vi "DAQ_OPC UA.vi"() -> (0 "Error Out":errorcluster)   [LabVIEW 2017]
uses:
  <vilib>/dex/Flush And Wait Empty Condition.ctl
  <vilib>/Platform/TimedLoop/XDataNode/timing_clust.ctl
  <vilib>/Platform/TimedLoop/XDataNode/nitl_modes.ctl
  <vilib>/Platform/TimedLoop/XDataNode/wakeup.ctl
  <vilib>/DAQmx/read.llb/DAQmx Read (Analog 1D DBL NChan 1Samp).vi
  <vilib>/DAQmx/miscellaneous.llb/DAQmx Fill In Error Info.vi
  <vilib>/Platform/TimedLoop/XDataNode/XDataNode.xnode
  <vilib>/Platform/TimedLoop/XDataNode/XDNodeRunTimeDep.lvlib
  <resource>/objmgr/ni.dex.rc
panel:
  out "Producer Loop Time":i64
  out "Consumer Loop Time":u32
  out "Time":dbl
  out "Available Elements for Writing":i32
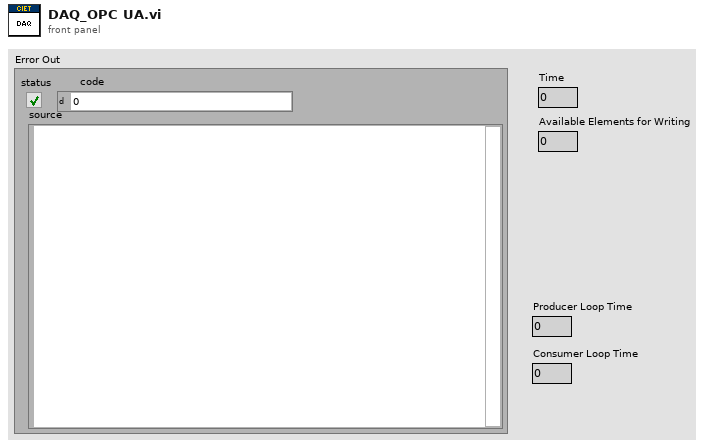
[diagram p1: front panel]
types:
  T1 = typedef "Flush And Wait Empty Condition.ctl" = u8
  T2 = typedef "XDNodeRunTimeDep.lvlib/timing_clust.ctl" = cluster{"Expected End [f-1]":u64, "Actual End [f-1]":u64, "Finished Late? [f-1]":bool, "Expected End [i-1]":u64, "Actual End [i-1]":u64, "Finished Late? [i-1]":bool, "Expected Start [i]":u64, "Actual Start [i]":u64, "Expected Start [f]":u64, "Actual Start [f]":u64, "Source Name":string, "Structure Name":string, "Period":i64, "Deadline":i64, "Offset":i64, "Start":i64, "Priority":i32, "Timeout":i32, "Mode":T3, "Wakeup Reason":T4, "Error":errorcluster, "Source Type":string, "Secondary Source Type":string, "Global End Time":u64, "Global Start Time":u64, "Frame Duration":u64, "Iteration Duration":u64, "Assigned CPU":i32, "I/O Scan Engine Mode":u32}
  T3 = typedef "XDNodeRunTimeDep.lvlib/nitl_modes.ctl" = enum32{"No Change", "Process missed periods, maintain original phase", "Discard missed periods, maintain original phase", "Process missed periods, ignore original phase", "Discard missed periods, ignore original phase"}
  T4 = typedef "XDNodeRunTimeDep.lvlib/wakeup.ctl" = enum32{"Normal", "Aborted", "Asynchronous wakeup", "Timing source error", "Timed loop error", "Timeout"}
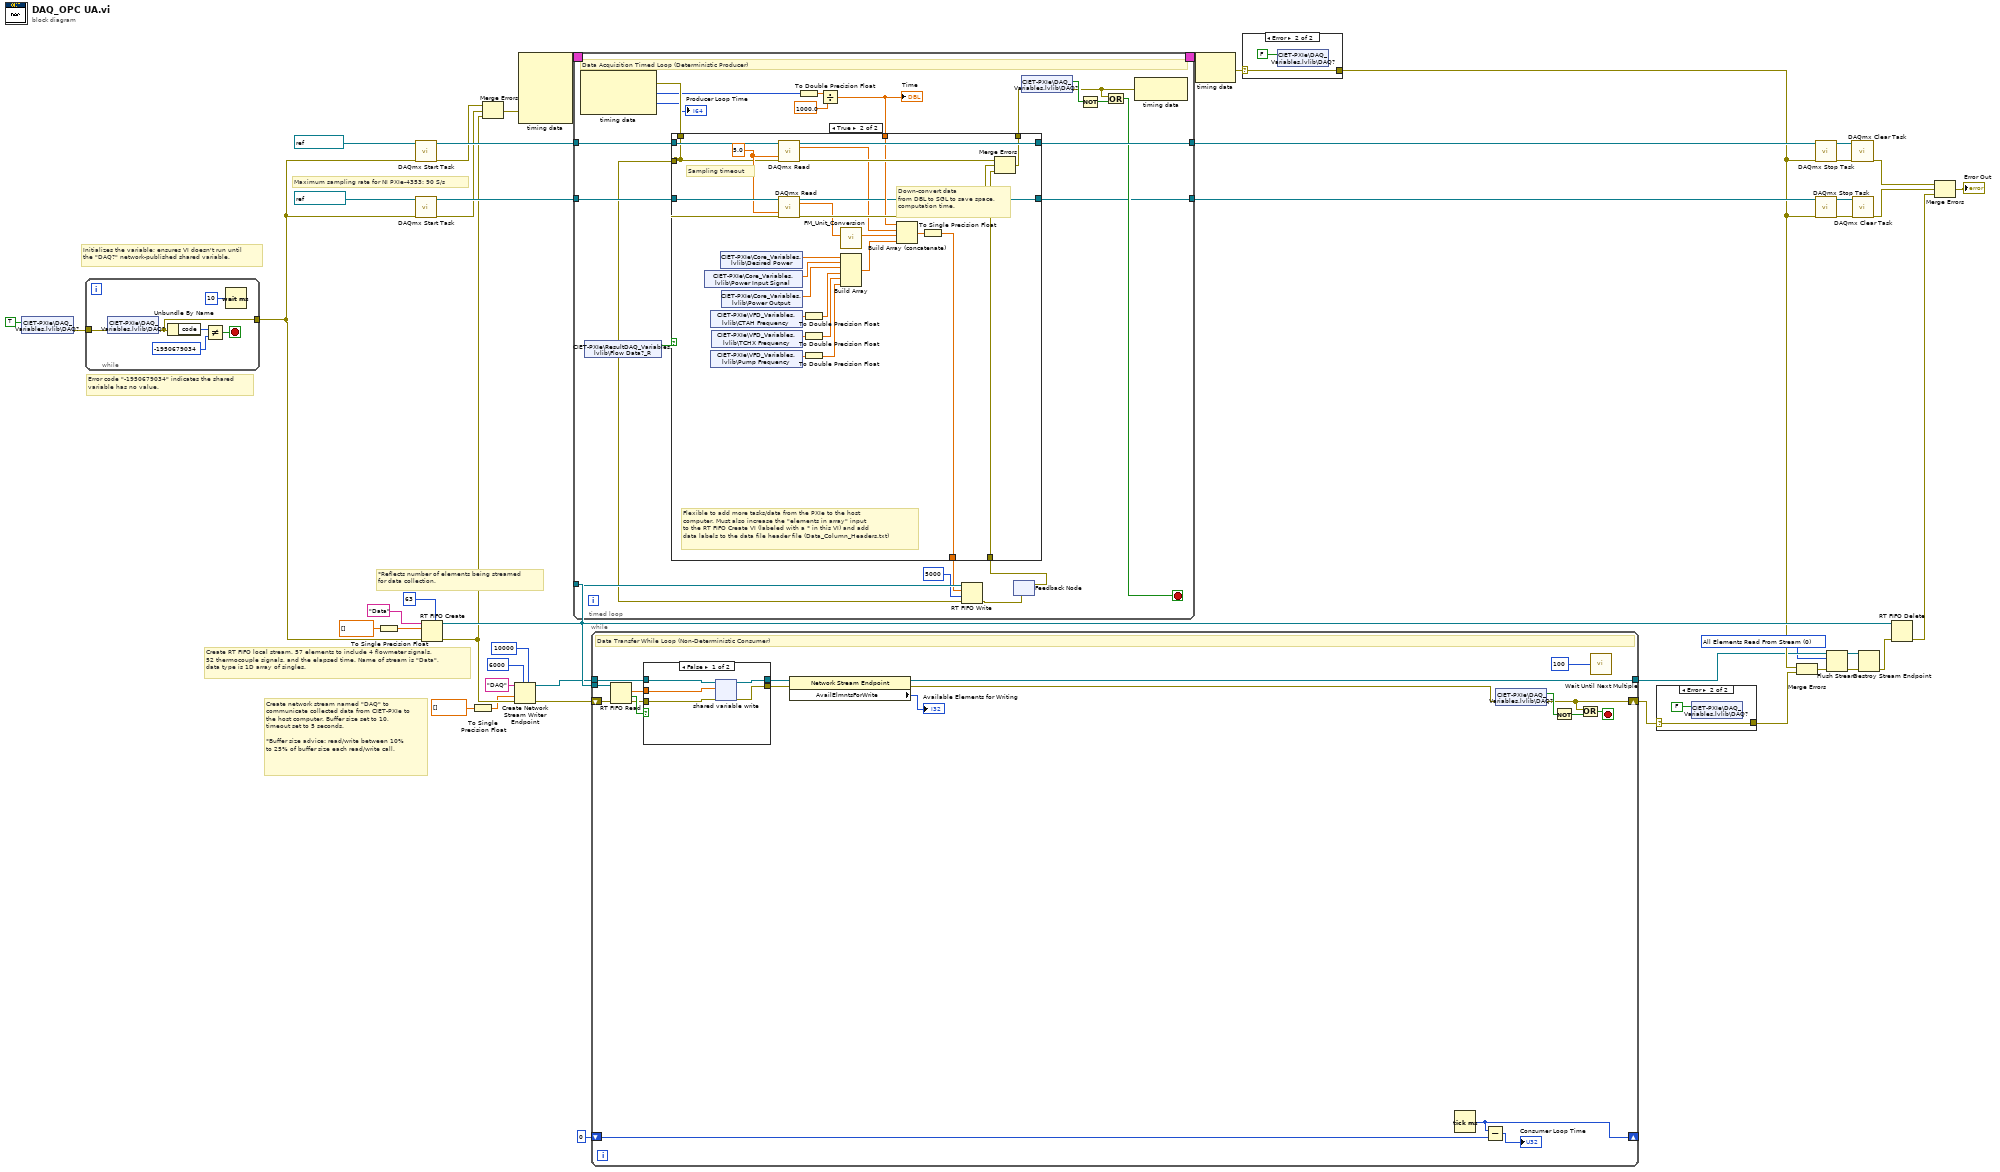
[diagram p0: block diagram]
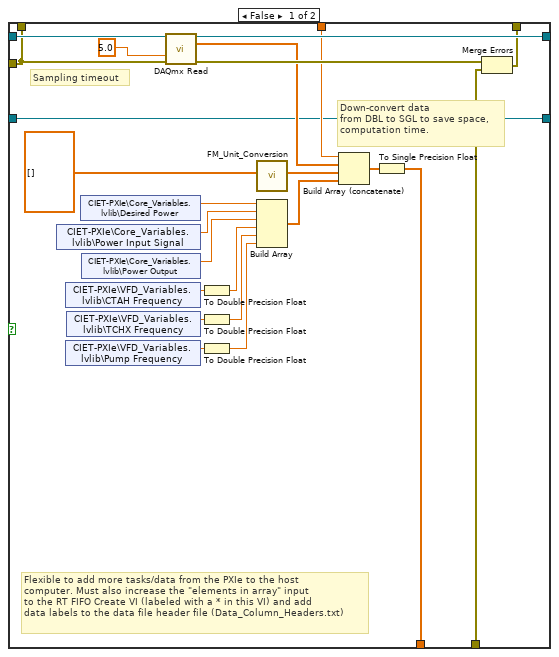
[diagram p5: hidden frame]
diagram:
  w2 = T1 0 items=["All Elements Read From Stream", "All Elements Available for Reading"] ("wait condition")
  # "*Reflects number of elements being streamed\nfor data collection."
  # "Create RT FIFO local stream. 57 elements to include 4 flowmeter signals,\n52 thermocouple signals, and the elapsed time. Name of stream is \"Data\",\ndata type is 1D array of singles."
  # "Create network stream named \"DAQ\" to communicate collected data from CIET-PXIe to the host computer. Buffer size set to 10, timeout set to 5 seconds. \n\n*Buffer size advice: read/write between 10%\nto 25% of buffer size each read/write call."
  # "Maximum sampling rate for NI PXIe-4353: 90 S/s"
  # "Initializes the variable; ensures VI doesn't run until\nthe \"DAQ?\" network-published shared variable."
  # "Error code \"-1950679034\" indicates the shared\nvariable has no value."
  n1 = shared-variable "CIET-PXIe\\DAQ_Variables.lvlib\\DAQ?"(TRUE ("Active?")) -> (error out=w22:errorcluster)  [unwired: 1 in]
  n2 = while {
    tunnel: w22 -> [w51]
    tunnel: [w50] -> w21
    stop <- w47 stop-if-true
    n3 = shared-variable "CIET-PXIe\\DAQ_Variables.lvlib\\DAQ?"(error in=w51) -> (error out=w50:errorcluster)  [unwired: 1 out]
    n4 = Unbundle By Name(w50) -> ("code"=w49:i32)
    n5 = Not Equal?(x=w49, y=-1950679034) -> (x != y?=w47:bool)
    n6 = Wait (ms)(milliseconds to wait=u32 10) -> ()  [unwired: 1 out]
  }
  n7 = To Single Precision Float(number=dbl[] []) -> (single precision float=w32:sgl[])
  n8 = call <vilib>:"DAQmx Start Task.vi"("task/channels in"=refnum<k21> "CIET-TC", "error in"=w21) -> ("task out"=w42:refnum<k21>, "error out"=w26:errorcluster)  [unwired: 12 in]
  n9 = call <vilib>:"DAQmx Start Task.vi"("task/channels in"=refnum<k21> "CIET-FM", "error in"=w21) -> ("task out"=w41:refnum<k21>, "error out"=w27:errorcluster)  [unwired: 12 in]
  n10 = RT FIFO Create(0:"Data" ("name (unnamed)"), 1:w32, 3:w21, 6:u32 63 ("elements in array (1)")) -> (8:w25:refnum<k33>, 11:w17:errorcluster)  [unwired: 4 in, 1 out]
  n11 = To Single Precision Float(number=dbl[] []) -> (single precision float=w7:sgl[])
  n12 = Merge Errors(w26, w27, w17) -> (w28:errorcluster)
  n13 = Create Network Stream Writer Endpoint(5:10000 ("timeout in ms (-1)"), 7:6000 ("writer buffer size"), 8:w17, 9:w7, 11:"DAQ" ("writer name")) -> (0:w18:errorcluster, 3:w16:refnum<k21>)  [unwired: 2 in]
  n14 = node-c288(w28) -> (w46:T2)  [unwired: 4 in]
  n15 = timed-loop {
    timing: w46 -> [_]
    timing-out: [_] -> w45
    tunnel: w25 -> [w71]
    tunnel: w42 -> [w74]
    tunnel: [w72] -> w36
    tunnel: w41 -> [w73]
    tunnel: [w59] -> w35
    stop <- w66 stop-if-true
    # "Data Acquisition Timed Loop (Deterministic Producer)"
    n16 = node-c288() -> (w69:errorcluster, w60:i64, →"Producer Loop Time":i64)  [unwired: 1 in]
    n17 = shared-variable "CIET-PXIe\\ResultDAQ_Variables.lvlib\\Flow Data?_R"() -> (w53:bool)  [unwired: 1 in, 1 out]
    n18 = To Double Precision Float(number=w60) -> (double precision float=w63:dbl)
    n19 = Divide(x=w63, y=1000.0) -> (x/y=w62:dbl)
    "Time" <- w62
    n20 = feedback #1() -> (w55:errorcluster)  [unwired: 1 in]
    n21 = case shown="True" w53 {
      tunnel: w74 -> [w98 w124]
      tunnel: w73 -> [w78 w123]
      tunnel: [w96 w121] -> w72
      tunnel: [w94 w119] -> w57
      tunnel: w69 -> [w75 w99]
      tunnel: w55 -> [w76 w116]
      tunnel: [w92 w115] -> w65
      tunnel: w62 -> [w91 w114]
      tunnel: [w78 w113] -> w59
      tunnel: [w75 w99] -> w54
      frame False {
        # "Flexible to add more tasks/data from the PXIe to the host \ncomputer. Must also increase the \"elements in array\" input \nto the RT FIFO Create VI (labeled with a * in this VI) and add\ndata labels to the data file header file (Data_Column_Headers.txt)"
        # "Down-convert data\nfrom DBL to SGL to save space,\ncomputation time."
        # "Sampling timeout"
        n22 = shared-variable "CIET-PXIe\\Core_Variables.lvlib\\Power Input Signal"() -> (w81:sgl)  [unwired: 1 in, 1 out]
        n23 = shared-variable "CIET-PXIe\\VFD_Variables.lvlib\\CTAH Frequency"() -> (w83:sgl)  [unwired: 1 in, 1 out]
        n24 = shared-variable "CIET-PXIe\\VFD_Variables.lvlib\\Pump Frequency"() -> (w85:sgl)  [unwired: 1 in, 1 out]
        n25 = shared-variable "CIET-PXIe\\VFD_Variables.lvlib\\TCHX Frequency"() -> (w84:sgl)  [unwired: 1 in, 1 out]
        n26 = shared-variable "CIET-PXIe\\Core_Variables.lvlib\\Desired Power"() -> (w80:sgl)  [unwired: 1 in, 1 out]
        n27 = shared-variable "CIET-PXIe\\Core_Variables.lvlib\\Power Output"() -> (w82:sgl)  [unwired: 1 in, 1 out]
        n28 = call-poly <vilib>:"DAQmx Read.vi"("task/channels in"=w98, "timeout"=5.0, "error in"=w75) -> ("task out"=w96:refnum<k21>, "data"=w90:dbl[], "error out"=w93:errorcluster)  [unwired: 10 in]
        n29 = To Double Precision Float(number=w83) -> (double precision float=w86:dbl)
        n30 = To Double Precision Float(number=w84) -> (double precision float=w87:dbl)
        n31 = To Double Precision Float(number=w85) -> (double precision float=w88:dbl)
        n32 = call "FM_Unit_Conversion.vi"("Input Array [A]"=dbl[] []) -> ("Output Array [kg/h]"=w89:dbl[])  [unwired: 10 in]
        n33 = Build Array(w80, w81, w82, w86, w87, w88) -> (w79:dbl[])
        n34 = Build Array (concatenate)(w91, w90, w89, w79) -> (w95:dbl[])
        n35 = To Single Precision Float(number=w95) -> (single precision float=w94:sgl[])
        n36 = Merge Errors(w93, w76) -> (w92:errorcluster)
      }
      frame True {
        w122 = 5.0 ("timeout")
        # "Flexible to add more tasks/data from the PXIe to the host \ncomputer. Must also increase the \"elements in array\" input \nto the RT FIFO Create VI (labeled with a * in this VI) and add\ndata labels to the data file header file (Data_Column_Headers.txt)"
        # "Down-convert data\nfrom DBL to SGL to save space,\ncomputation time."
        # "Sampling timeout"
        n37 = shared-variable "CIET-PXIe\\Core_Variables.lvlib\\Power Input Signal"() -> (w102:sgl)  [unwired: 1 in, 1 out]
        n38 = shared-variable "CIET-PXIe\\VFD_Variables.lvlib\\CTAH Frequency"() -> (w104:sgl)  [unwired: 1 in, 1 out]
        n39 = shared-variable "CIET-PXIe\\VFD_Variables.lvlib\\Pump Frequency"() -> (w106:sgl)  [unwired: 1 in, 1 out]
        n40 = shared-variable "CIET-PXIe\\VFD_Variables.lvlib\\TCHX Frequency"() -> (w105:sgl)  [unwired: 1 in, 1 out]
        n41 = shared-variable "CIET-PXIe\\Core_Variables.lvlib\\Desired Power"() -> (w101:sgl)  [unwired: 1 in, 1 out]
        n42 = shared-variable "CIET-PXIe\\Core_Variables.lvlib\\Power Output"() -> (w103:sgl)  [unwired: 1 in, 1 out]
        n43 = call-poly <vilib>:"DAQmx Read.vi"("task/channels in"=w124, "timeout"=w122, "error in"=w99) -> ("task out"=w121:refnum<k21>, "data"=w112:dbl[], "error out"=w117:errorcluster)  [unwired: 10 in]
        n44 = call-poly <vilib>:"DAQmx Read.vi"("task/channels in"=w123, "timeout"=w122, "error in"=w99) -> ("task out"=w113:refnum<k21>, "data"=w110:dbl[], "error out"=w118:errorcluster)  [unwired: 10 in]
        n45 = To Double Precision Float(number=w104) -> (double precision float=w107:dbl)
        n46 = To Double Precision Float(number=w105) -> (double precision float=w108:dbl)
        n47 = To Double Precision Float(number=w106) -> (double precision float=w109:dbl)
        n48 = call "FM_Unit_Conversion.vi"("Input Array [A]"=w110) -> ("Output Array [kg/h]"=w111:dbl[])  [unwired: 10 in]
        n49 = Build Array(w101, w102, w103, w107, w108, w109) -> (w100:dbl[])
        n50 = Build Array (concatenate)(w114, w112, w111, w100) -> (w120:dbl[])
        n51 = To Single Precision Float(number=w120) -> (single precision float=w119:sgl[])
        n52 = Merge Errors(w117, w118, w116) -> (w115:errorcluster)
      }
    }
    n53 = RT FIFO Write(0:w71, 1:w57, 2:5000 ("timeout in ms (0)"), 3:w54) -> (11:w56:errorcluster)  [unwired: 1 in, 3 out]
    n54 = feedback-in #1(w56) -> ()
    n55 = shared-variable "CIET-PXIe\\DAQ_Variables.lvlib\\DAQ?"(error in=w65) -> (w68:bool, error out=w64:errorcluster)
    n56 = Not(x=w68) -> (.not. x?=w67:bool)
    n57 = Or(x=w64, y=w67) -> (x .or. y?=w66:bool)
    n58 = node-c288(w64) -> ()  [unwired: 1 out]
  }
  n59 = while {
    tunnel: w25 -> [w150]
    shift-right: [w139] -> w19
    shift-left: w18 -> [w149]
    tunnel: w16 -> [w141]
    tunnel: [w136] -> w9
    shift-right: [w134] -> _
    shift-left: u32 0 ("millisecond timer value") -> [w133]
    stop <- w142 stop-if-true
    # "Data Transfer While Loop (Non-Deterministic Consumer)"
    n60 = RT FIFO Read(0:w150, 3:w149) -> (9:w146:sgl[], 10:w147:bool, 11:w145:errorcluster)  [unwired: 2 in, 2 out]
    n61 = case shown="False" w147 {
      tunnel: w146 -> [w151 _]
      tunnel: w145 -> [w155 w157]
      tunnel: [w154 w157] -> w138
      tunnel: w141 -> [w153 w156]
      tunnel: [w152 w156] -> w137
      frame False {
        n62 = shared-variable-write(w153, w155, w151) -> (w152:refnum<k21>, w154:errorcluster)  [unwired: 1 in, 1 out]
      }
      frame True {
      }
    }
    n63 = property class="Network Stream Endpoint"(reference=w137, error in=w138) -> (reference out=w136:refnum<k21>, error out=w135:errorcluster, "AvailElmntsForWrite"=→"Available Elements for Writing":i32)
    n64 = Tick Count (ms)() -> (millisecond timer value=w134:u32)
    n65 = Subtract(x=w134, y=w133) -> (x-y=→"Consumer Loop Time":u32)
    n66 = shared-variable "CIET-PXIe\\DAQ_Variables.lvlib\\DAQ?"(error in=w135) -> (w144:bool, error out=w139:errorcluster)
    n67 = Not(x=w144) -> (.not. x?=w143:bool)
    n68 = Or(x=w139, y=w143) -> (x .or. y?=w142:bool)
    n69 = call "Wait Until Next Multiple"("Count(mSec)"=u32 100) -> ()  [unwired: 1 out]
  }
  n70 = node-c288(w45) -> (w20:errorcluster)
  n71 = case shown="Error" w20 {
    selector: w20 -> [w158 w159]
    tunnel: [w158 w159] -> w15
    frame No Error {
    }
    frame Error {
      n72 = shared-variable "CIET-PXIe\\DAQ_Variables.lvlib\\DAQ?"(FALSE ("DAQ?")) -> ()  [unwired: 1 in, 1 out]
    }
  }
  n73 = case shown="Error" w19 {
    selector: w19 -> [w161 w162]
    tunnel: [w161 w162] -> w14
    frame No Error {
    }
    frame Error {
      n74 = shared-variable "CIET-PXIe\\DAQ_Variables.lvlib\\DAQ?"(FALSE ("DAQ?")) -> ()  [unwired: 1 in, 1 out]
    }
  }
  n75 = Merge Errors(w15, w14) -> (w11:errorcluster)
  n76 = call <vilib>:"DAQmx Stop Task.vi"("task/channels in"=w36, "error in"=w15) -> ("task out"=w39:refnum<k21>, "error out"=w40:errorcluster)  [unwired: 12 in]
  n77 = call <vilib>:"DAQmx Stop Task.vi"("task/channels in"=w35, "error in"=w15) -> ("task out"=w37:refnum<k21>, "error out"=w38:errorcluster)  [unwired: 12 in]
  n78 = Flush Stream(8:w11, 10:w2, 11:w9) -> (0:w13:errorcluster, 3:w12:refnum<k21>)  [unwired: 1 in, 1 out]
  n79 = call <vilib>:"DAQmx Clear Task.vi"("task in"=w39, "error in"=w40) -> ("error out"=w34:errorcluster)  [unwired: 13 in]
  n80 = call <vilib>:"DAQmx Clear Task.vi"("task in"=w37, "error in"=w38) -> ("error out"=w33:errorcluster)  [unwired: 13 in]
  n81 = Destroy Stream Endpoint(8:w13, 11:w12) -> (0:w10:errorcluster)
  n82 = RT FIFO Delete(0:w25, 3:w10) -> (11:w4:errorcluster)  [unwired: 1 in]
  n83 = Merge Errors(w34, w33, w4) -> (→"Error Out":errorcluster)
